vi "ReadallDevicesv1.vi"(0 "GPIB HP 2":string="13", 1 "LI 3":bool, 2 "LI 2":bool, 3 "LI 1":bool, 4 "Nr. of Accumulations":i32=5, 5 "HP 2":bool, 7 "GPIB HP":string="14", 8 "Y-Axis Field (kG)":dbl, 9 "HP 1":bool=TRUE, 10 "Radial (r) Field (kG) 2":dbl, 11 "error in":T1, 12 "GPIB L 3":string="8", 13 "GPIB L 2":string="8", 14 "GPIB L 1":string="8") -> (6 "appended array":dbl[](array[numeric]), 15 "error out":errorcluster)   [LabVIEW 2009]
panel:
  out "Messfile Refnum":refnum<file>
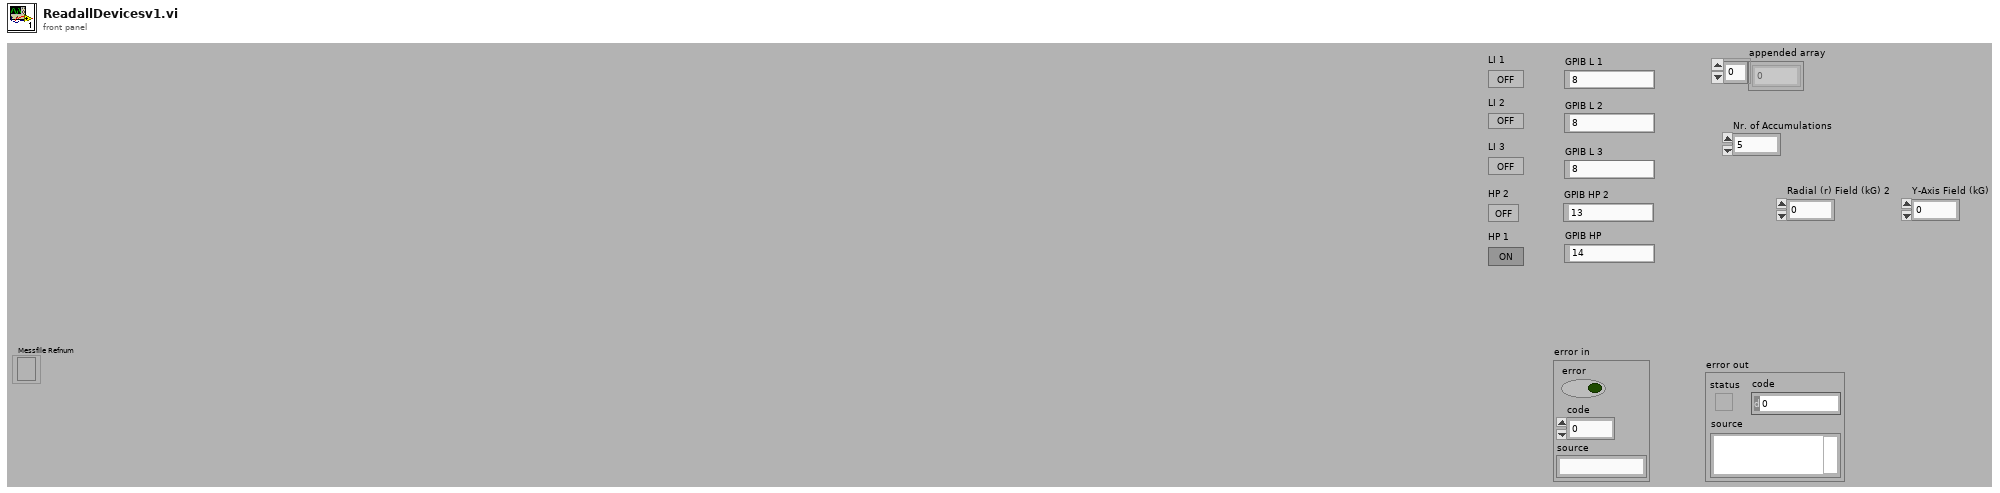
[diagram p1: front panel]
types:
  T1 = cluster{"error":bool, "code":i32, "source":string}
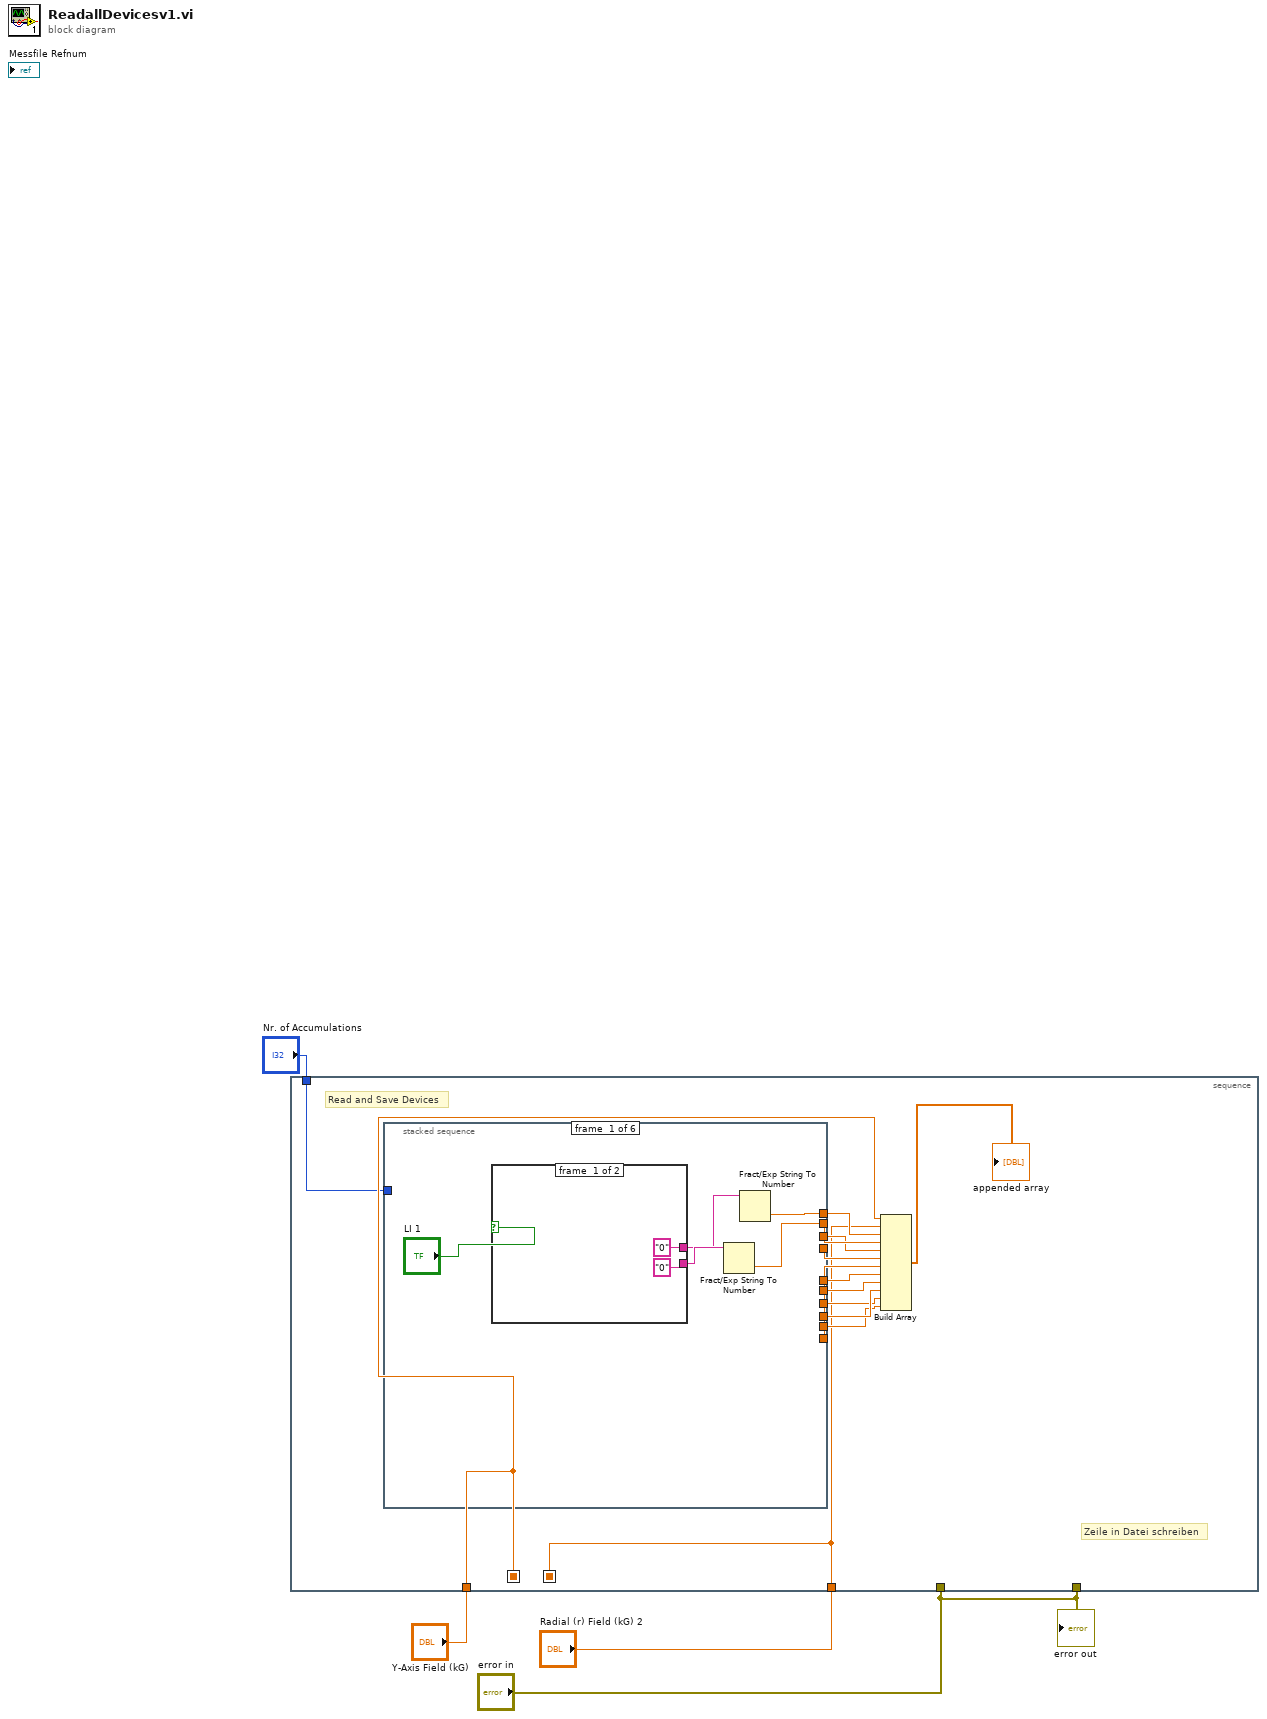
[diagram p0: block diagram]
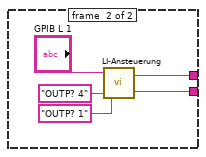
[diagram p2: hidden frame]
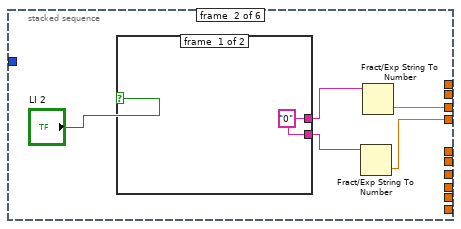
[diagram p3: hidden frame]
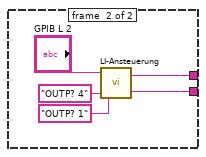
[diagram p4: hidden frame]
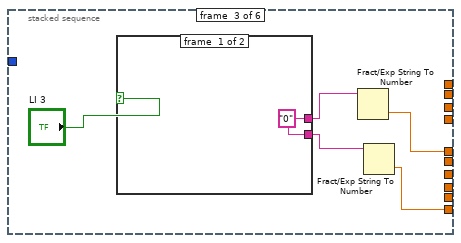
[diagram p5: hidden frame]
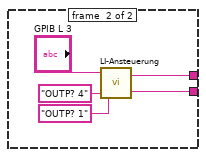
[diagram p6: hidden frame]
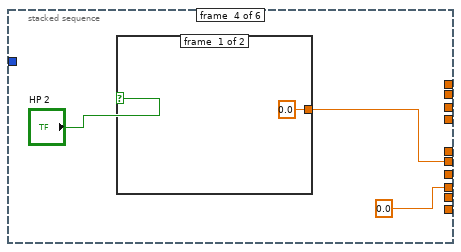
[diagram p7: hidden frame]
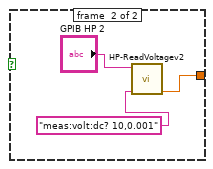
[diagram p8: hidden frame]
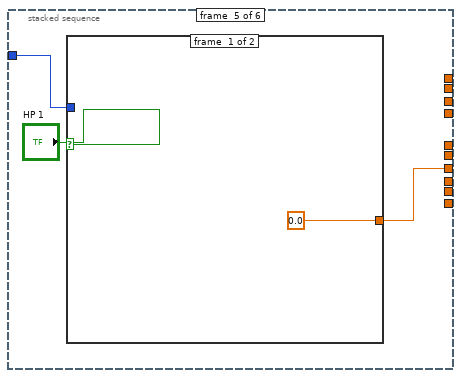
[diagram p9: hidden frame]
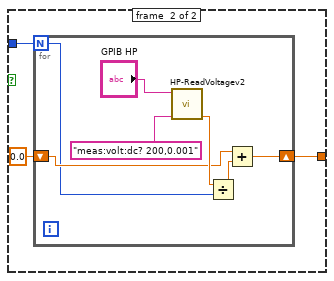
[diagram p10: hidden frame]
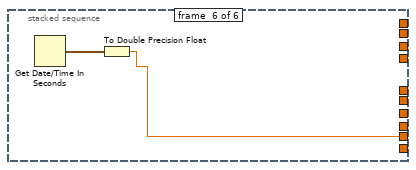
[diagram p11: hidden frame]
diagram:
  n1 = stacked-sequence {
    seq-local: [w6] -> [_]
    seq-local: [w7] -> [_]
    tunnel: "error in" -> [_]
    tunnel: "Y-Axis Field (kG)" -> [w7]
    tunnel: "Radial (r) Field (kG) 2" -> [w6]
    tunnel: "error in" -> [_]
    tunnel: "Nr. of Accumulations" -> [w5]
    frame #0 {
      # "Zeile in Datei schreiben"
      # "Read and Save Devices"
      n2 = stacked-sequence {
        tunnel: [w20 _ _ _ _ _] -> w18
        tunnel: [w19 _ _ _ _ _] -> w17
        tunnel: [_ w33 _ _ _ _] -> w16
        tunnel: [_ w31 _ _ _ _] -> w15
        tunnel: [_ _ w43 _ _ _] -> w14
        tunnel: [_ _ w42 _ _ _] -> w13
        tunnel: [_ _ _ w54 _ _] -> w12
        tunnel: [_ _ _ 0.0 _ _] -> w11
        tunnel: [_ _ _ _ w61 _] -> w10
        tunnel: [_ _ _ _ _ w74] -> w9
        tunnel: w5 -> [_ _ _ _ w60 _]
        frame #0 {
          n3 = case shown="True" "LI 1" {
            tunnel: ["0" ("Antwort2") w27] -> w22
            tunnel: ["0" ("Antwort1") w26] -> w21
            frame #0 {
            }
            frame #1 {
              n4 = call "LI-Ansteuerung.vi"("Frage2"="OUTP? 4", "Frage1"="OUTP? 1", "address string"="GPIB L 1") -> ("Antwort2"=w27:string, "Antwort1"=w26:string)
            }
          }
          n5 = Fract/Exp String To Number(string=w22) -> (number=w19:dbl)  [unwired: 3 in, 1 out]
          n6 = Fract/Exp String To Number(string=w21) -> (number=w20:dbl)  [unwired: 3 in, 1 out]
        }
        frame #1 {
          n7 = case shown="False" "LI 2" {
            tunnel: [w36 w38] -> w32
            tunnel: [w36 w37] -> w34
            frame #0 {
              w36 = "0" ("Antwort1")
            }
            frame #1 {
              n8 = call "LI-Ansteuerung.vi"("Frage2"="OUTP? 4", "Frage1"="OUTP? 1", "address string"="GPIB L 2") -> ("Antwort2"=w38:string, "Antwort1"=w37:string)
            }
          }
          n9 = Fract/Exp String To Number(string=w32) -> (number=w31:dbl)  [unwired: 3 in, 1 out]
          n10 = Fract/Exp String To Number(string=w34) -> (number=w33:dbl)  [unwired: 3 in, 1 out]
        }
        frame #2 {
          n11 = case shown="False" "LI 3" {
            tunnel: [w47 w49] -> w44
            tunnel: [w47 w48] -> w45
            frame #0 {
              w47 = "0" ("Antwort1")
            }
            frame #1 {
              n12 = call "LI-Ansteuerung.vi"("Frage2"="OUTP? 4", "Frage1"="OUTP? 1", "address string"="GPIB L 3") -> ("Antwort2"=w49:string, "Antwort1"=w48:string)
            }
          }
          n13 = Fract/Exp String To Number(string=w45) -> (number=w43:dbl)  [unwired: 3 in, 1 out]
          n14 = Fract/Exp String To Number(string=w44) -> (number=w42:dbl)  [unwired: 3 in, 1 out]
        }
        frame #3 {
          n15 = case shown="False" "HP 2" {
            tunnel: [0.0 ("Voltage") w57] -> w54
            frame #0 {
            }
            frame #1 {
              n16 = call "HP-ReadVoltagev2.vi"("String"="meas:volt:dc? 10,0.001", "HP-Mulitmeter\nGPIB Address"="GPIB HP 2") -> ("Voltage"=w57:dbl)  [unwired: 9 in]
            }
          }
        }
        frame #4 {
          n17 = case shown="True" "HP 1" {
            tunnel: [0.0 ("Voltage") w66] -> w61
            tunnel: w60 -> [_ w65]
            frame #0 {
            }
            frame #1 {
              n18 = for {
                N: w65 -> [w67]
                shift-right: [w69] -> w66
                shift-left: 0.0 -> [w68]
                n19 = call "HP-ReadVoltagev2.vi"("String"="meas:volt:dc? 200,0.001", "HP-Mulitmeter\nGPIB Address"="GPIB HP") -> ("Voltage"=w71:dbl)  [unwired: 9 in]
                n20 = Divide(x=w71, y=w67) -> (x/y=w70:dbl)
                n21 = Add(x=w68, y=w70) -> (x+y=w69:dbl)
              }
            }
          }
        }
        frame #5 {
          n22 = Get Date/Time In Seconds() -> (seconds since 1Jan1904=w75:timestamp)
          n23 = To Double Precision Float(number=w75) -> (double precision float=w74:dbl)
        }
      }
      n24 = Build Array(w7, w6, w18, w17, w16, w15, w13, w14, w12, w11, w10, w9) -> (→"appended array":dbl[])
    }
  }
  "error out" <- "error in"
